vi "Filament Control.vi"(8 "error in (no error)":errorcluster, 9 "Filament":bool, 10 "Filament ID":i32, 11 "Lesker Pressure in":refnum<class "Lesker Pressure.lvclass">) -> (0 "error out":errorcluster, 3 "Lesker Pressure out":refnum<class "Lesker Pressure.lvclass">)   [LabVIEW 2024, in "Lesker Pressure.lvclass"]
uses:
  Lesker Pressure.lvclass
  Lesker Pressure.lvclass/Lesker Pressure.ctl
  Pressure Monitor.lvclass
panel:
  out "Response":string="*01 2.89E-04\r"
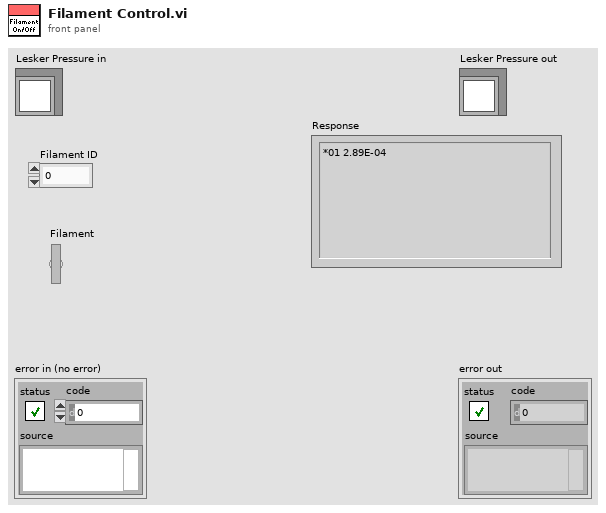
[diagram p1: front panel]
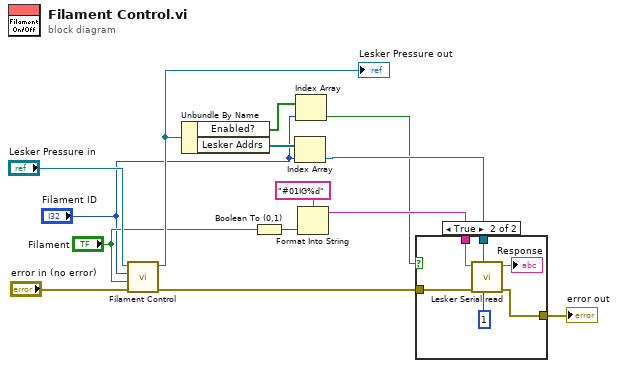
[diagram p0: block diagram]
diagram:
  n1 = call-parent "Filament Control.vi"("error in (no error)"="error in (no error)", "Filament"="Filament", "Filament ID"="Filament ID", "Pressure Monitor in"="Lesker Pressure in") -> ("error out"=w5:errorcluster, "Pressure Monitor out"=w12:refnum<class "Lesker Pressure.lvclass">)  [unwired: 6 in]
  "Lesker Pressure out" <- w12
  n2 = Unbundle By Name(w12) -> ("Enabled?"=w3:bool[], "Lesker Addrs"=w11:refnum<visa-resource-name>[])
  n3 = Boolean To (0,1)(Boolean="Filament") -> (0, 1=w8:i16)
  n4 = Index Array(array=w11, index="Filament ID") -> (element=w10:refnum<visa-resource-name>)
  n5 = Index Array(array=w3, index="Filament ID") -> (element=w1:bool)
  n6 = Format Into String(format string="#01IG%d", w8) -> (resulting string=w6:string)  [unwired: 2 in, 1 out]
  n7 = case shown="True" w1 {
    tunnel: w10 -> [_ w21]
    tunnel: w6 -> [_ w20]
    tunnel: w5 -> [w15 w18]
    tunnel: [w15 w17] -> w4
    frame False {
    }
    frame True {
      n8 = call "Lesker Serial read.vi"("Number of reads"=1, "VISA resource name"=w21, "error in (no error)"=w18, "Command"=w20) -> ("error out"=w17:errorcluster, "Response"=→"Response":string)  [unwired: 5 in, 1 out]
    }
  }
  "error out" <- w4
